vi "CRYSave Virtual Data.vi"(8 "error in":errorcluster) -> (0 "error out":errorcluster)   [LabVIEW 2013]
uses:
  CRYMisc vis settings global.vi
  CRYMainGlobal.vi
panel:
  # "Virtual Data Saving"
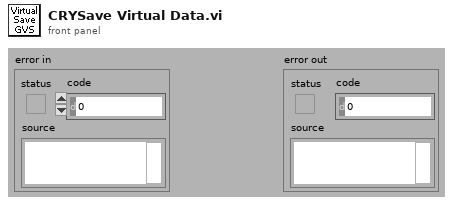
[diagram p1: front panel]
types:
  T1 = cluster{"Sinal Gen":string, "RTA":string, "Scope-FFT":string, "Voltmeter":string}
  T2 = cluster{"gen'r mode":i32, "frequency":u32, "output level":dbl, "wave path":string, "wav play mode":i32, "duration":dbl, "n times":i32, "channel":i32, "wav level":dbl, "EQ":bool, "f knob log":bool, "f knob low":dbl, "f knob high":dbl, "ol knob log":bool, "ol knob low":dbl, "ol knob high":dbl, "Lin Display Prefs":string, "dB Display Prefs":string, "Duration noise":dbl, "Min freq noise":dbl, "Max freq noise":dbl, "Signal Type":string, "Play Sine Wave":i32}
  T3 = typedef "CRYScope-FFT.ctl" = cluster{"window":i32, "n avgs":i32, "lin/exp avg":i32, "pwr/cplx avg":i32, "time (ms)":dbl, "fft lines":i32, "scope/fft mode":i32, "channel":i32, "trig. channel":i32, "Applay Correction":bool, "Time Display":string, "Freq. Weighting":string, "Ave/Max/Min":u16, "Trigger Level":dbl, "Trigger Unit":u16, "Trigger Time Offset":dbl, "Trigger Slope":u16, "Trigger/Free Run":bool, "continuous":bool, "Spectrum Display":string, "Calc FFT":bool, "Y-axis":string, "Signal Type":string}
  T4 = typedef "CRYMultimeter.ctl" = cluster{"Ave/Max/Min":i32, "Level":i32, "Channel":i32, "Signal Type":string, "Weighting":string, "Applay Correction":bool, "lin/exp avg":u16, "rec time (sec)":dbl, "Average Time (Sec)":dbl, "Lin Display Prefs":string, "dB Display Prefs":string, "Time Weighting":u16, "Display":u16}
  T5 = cluster{"octave":i32, "det time":i32, "det sec":dbl, "lin/exp":i32, "weighting":i32, "channel":i32, "Ave/Max/Min":u16, "continuous":bool, "Applay Correction":bool, "Display":u16, "Signal Type":string}
  T6 = enum16{"open", "replace", "create", "open or create", "replace or create", "replace or create with confirmation"}
  T7 = enum16{"big-endian, network order", "native, host order", "little-endian"}
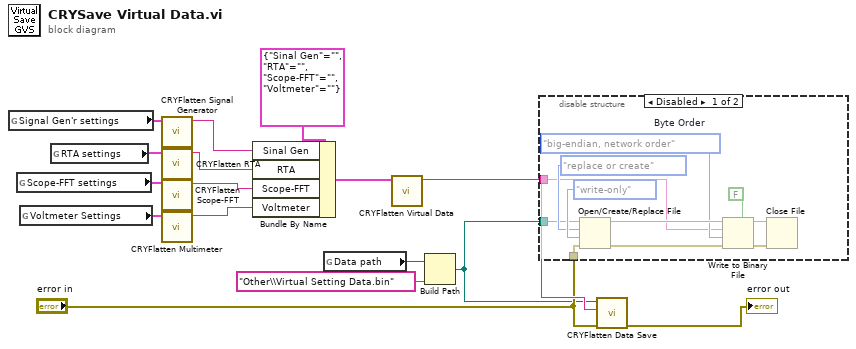
[diagram p0: block diagram]
diagram:
  n1 = global read "CRYMisc vis settings global.vi" "Signal Gen'r settings"() -> (w14:T2)
  n2 = global read "CRYMisc vis settings global.vi" "Scope-FFT settings"() -> (w10:T3)
  n3 = global read "CRYMisc vis settings global.vi" "Voltmeter Settings"() -> (w12:T4)
  n4 = global read "CRYMisc vis settings global.vi" "RTA settings"() -> (w11:T5)
  n5 = call "CRYFlatten Signal Generator.vi"("Signal Gen'r settings"=w14) -> ("Flat Signal Gen'r settings"=w13:string)  [unwired: 10 out]
  n6 = call "CRYFlatten RTA.vi"("RTA settings"=w11) -> ("Flat RTA settings"=w8:string)  [unwired: 10 out]
  n7 = call "CRYFlatten Scope-FFT.vi"("Scope-FFT settings"=w10) -> ("Flat Scope-FFT settings"=w9:string)  [unwired: 10 out]
  n8 = call "CRYFlatten Multimeter.vi"("Voltmeter Settings"=w12) -> ("Flat Voltmeter setup"=w7:string)  [unwired: 10 out]
  n9 = Bundle By Name(cluster=T1 {"Sinal Gen"="", "RTA"="", "Scope-FFT"="", "Voltmeter"=""}, "Sinal Gen"=w13, "RTA"=w8, "Scope-FFT"=w9, "Voltmeter"=w7) -> (w15:T1)
  n10 = global read "CRYMainGlobal.vi" "Data path"() -> (w2:path)
  n11 = call "CRYFlatten Virtual Data.vi"("Virtual cluster"=w15) -> ("Flat Virtual Settings"=w6:string)  [unwired: 10 out]
  n12 = Build Path(base path=w2, name or relative path="Other\\Virtual Setting Data.bin") -> (appended path=w1:path)
  n13 = disable-structure shown="Disabled" {
    disable-tunnel: w1 -> [w19 _]
    disable-tunnel: w6 -> [w18 _]
    disable-tunnel: "error in" -> [w17 _]
    frame Disabled {
      w24 = T7."big-endian, network order"  # Byte Order
      n14 = Open/Create/Replace File(file path (use dialog)=w19, error in=w17, operation (0:open)=T6."replace or create", access (0:read/write)=enum16{"read/write", "read-only", "write-only"}."write-only") -> (refnum out=w27:refnum<file>, error out=w21:errorcluster)  [unwired: 3 out]
      n15 = Write to Binary File(file (use dialog)=w27, data=w18, error in=w21, 5:FALSE ("prepend array or string size? (T)"), 9:w24) -> (refnum out=w22:refnum<file>, error out=w20:errorcluster)  [unwired: 2 out]
      n16 = Close File(refnum=w22, error in=w20) -> ()  [unwired: 2 out]
    }
    frame Enabled {
    }
  }
  n17 = call "CRYFlatten Data Save.vi"("error in"="error in", "Any Flatten Data"=w6, "Path In"=w1) -> ("error out"=→"error out":errorcluster)  [unwired: 5 in, 1 out]
